vi "Initialize Hardware References.vi"(6 "error in (no error)":errorcluster, 8 "Acq Settings in":T9 {"Config Settings"."Simulated Sensor Injection" scale=0.0..100.0}, 9 "Stimulus Settings in":T1) -> (0 "error out":errorcluster, 2 "Stimulus Task":refnum<k21>, 3 "Calibration Task":refnum<k21>)   [LabVIEW 2026, in "Acquisition.lvlib"]
doc: "Initialize the hardware references."
uses:
  Acquisition.lvlib
  controls/UI/Acq Settings.ctl
  Instrument Specifications Configuration.ctl
  Instrument Specifications Cluster Configuration.ctl
  controls/UI/Measurement Role.ctl
  controls/UI/Config Settings.ctl
  controls/Controller/Stimulus Settings.ctl
  controls/Controller/Stimulus Outputs.ctl
  controls/Controller/Stimulus Output.ctl
  controls/Controller/Controller Core Data.ctl
  controls/UI/Units Enum.ctl
  controls/UI/Signal Enum.ctl
  controls/Controller/Stimulus Output Configuration.ctl
  controls/Controller/Stimulus Role.ctl
  Settings/Settings.lvlib
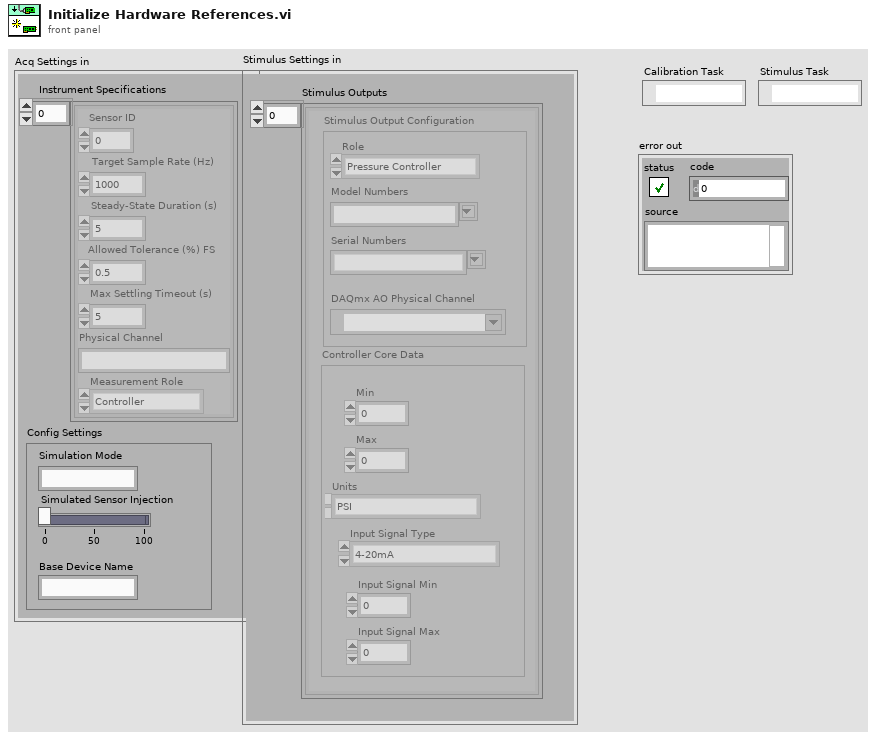
[diagram p1: front panel]
types:
  T1 = typedef "Settings.lvlib/Stimulus Settings.ctl" = cluster{"Stimulus Outputs":T2}
  T2 = typedef "Settings.lvlib/Stimulus Outputs.ctl" = T3[]
  T3 = typedef "Settings.lvlib/Stimulus Output.ctl" = cluster{"Controller Core Data":T4, "Stimulus Output Configuration":T7}
  T4 = typedef "Settings.lvlib/Controller Core Data.ctl" = cluster{"Min":dbl, "Max":dbl, "Units":T5, "Input Signal Type":T6, "Input Signal Min":dbl, "Input Signal Max":dbl}
  T5 = typedef "Units Enum.ctl" = enum16{"PSI", "Deg C", "kPa", "GPM"}
  T6 = typedef "Signal Enum.ctl" = enum16{"4-20mA", "0-10V", "Thermocouple Type K"}
  T7 = typedef "Settings.lvlib/Stimulus Output Configuration.ctl" = cluster{"DAQmx AO Physical Channel":tag, "Role":T8, "Model Numbers":string, "Serial Numbers":string}
  T8 = typedef "Stimulus Role.ctl" = enum16{"Pressure Controller", "Temperature Controller"}
  T9 = typedef "Acq Settings.ctl" = cluster{"Instrument Specifications":T10, "Config Settings":T13}
  T10 = typedef "Acquisition.lvlib/Instrument Specifications Configuration.ctl" = T11[]
  T11 = typedef "Acquisition.lvlib/Instrument Specifications Cluster Configuration.ctl" = cluster{"Sensor ID":i32, "Target Sample Rate (Hz)":dbl, "Steady-State Duration (s)":i32, "Allowed Tolerance (%) FS":dbl, "Max Settling Timeout (s)":i32, "Physical Channel":string, "Measurement Role":T12}
  T12 = typedef "Settings.lvlib/Measurement Role.ctl" = enum16{"Controller", "Reference", "UUT", "Disable", "All"}
  T13 = typedef "Config Settings.ctl" = cluster{"Simulated Sensor Injection":dbl, "Base Device Name":string, "Simulation Mode":string}
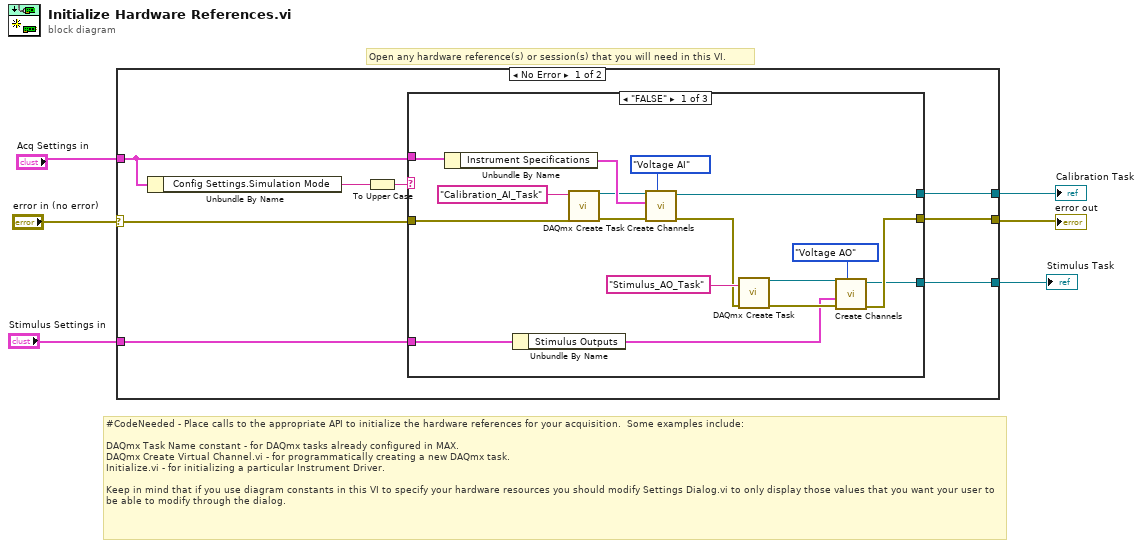
[diagram p0: block diagram]
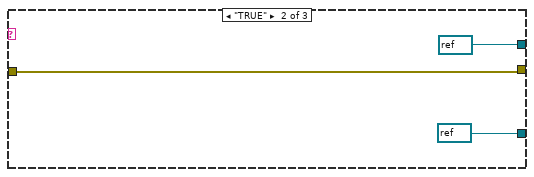
[diagram p2: hidden frame]
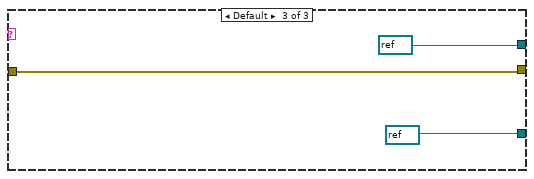
[diagram p3: hidden frame]
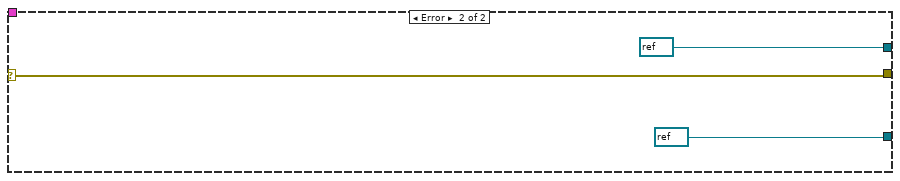
[diagram p4: hidden frame]
diagram:
  # "Open any hardware reference(s) or session(s) that you will need in this VI."
  # "#CodeNeeded - Place calls to the appropriate API to initialize the hardware references for your acquisition.  Some examples include:\n\nDAQmx Task Name constant - for DAQmx tasks already configured in MAX.\nDAQmx Create Virtual Channel.vi - for programmatically creating a new DAQmx task.\nInitialize.vi - for initializing a particular Instrument Driver.\n\nKeep in mind that if you use diagram constants in this VI to specify your hardware resources you should modify Settings Dialog.vi to only display those values that you want your user to be able to modify through the dialog."
  n1 = case shown="No Error" "error in (no error)" {
    selector: "error in (no error)" -> [w13 w40]
    tunnel: [w7 w40] -> w5
    tunnel: "Acq Settings in" -> [w12 _]
    tunnel: [w14 refnum<k21> refnum ("task out")] -> w3
    tunnel: "Stimulus Settings in" -> [w9 _]
    tunnel: [w8 refnum<k21> refnum ("task out")] -> w1
    frame No Error {
      n2 = Unbundle By Name(w12) -> ("Config Settings.Simulation Mode"=w11:string)
      n3 = To Upper Case(1:w11) -> (0:w10:string)
      n4 = case shown="\"FALSE\"" w10 {
        tunnel: w12 -> [w31 _ _]
        tunnel: [w17 w33 w36] -> w7
        tunnel: [w30 refnum<k21> refnum ("task out") refnum<k21> refnum ("task out")] -> w14
        tunnel: w13 -> [w24 w33 w36]
        tunnel: w9 -> [w25 _ _]
        tunnel: [w16 refnum<k21> refnum ("task out") refnum<k21> refnum ("task out")] -> w8
        frame "FALSE" {
          n5 = Unbundle By Name(w31) -> ("Instrument Specifications"=w29:T10)
          n6 = Unbundle By Name(w25) -> ("Stimulus Outputs"=w15:T2)
          n7 = call <vilib>:"DAQmx Create Task.vi"("new task name"="Calibration_AI_Task", "error in"=w24) -> ("task out"=w28:refnum<k21>, "error out"=w19:errorcluster)  [unwired: 12 in]
          n8 = call "Create Channels.vi"("I/O Type"=enum16{"Voltage AO", "Voltage AI"}."Voltage AI", "error in (no error)"=w19, "Instrument Specifications"=w29, "Refnum in"=w28) -> ("error out"=w22:errorcluster, "Refnum out"=w30:refnum<k21>)  [unwired: 6 in]
          n9 = call <vilib>:"DAQmx Create Task.vi"("new task name"="Stimulus_AO_Task", "error in"=w22) -> ("task out"=w20:refnum<k21>, "error out"=w21:errorcluster)  [unwired: 12 in]
          n10 = call "Create Channels.vi"("I/O Type"=enum16{"Voltage AO", "Voltage AI"}."Voltage AO", "error in (no error)"=w21, "Stimulus Outputs"=w15, "Refnum in"=w20) -> ("error out"=w17:errorcluster, "Refnum out"=w16:refnum<k21>)  [unwired: 6 in]
        }
        frame "TRUE" {
        }
        frame Default {
        }
      }
    }
    frame Error {
    }
  }
  "error out" <- w5
  "Calibration Task" <- w3
  "Stimulus Task" <- w1
